vi "TDMS Strip Illegal Characters.vi"(5 "String":string) -> (2 "Legal String":string)   [LabVIEW 2011]
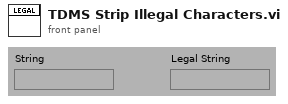
[diagram p1: front panel]
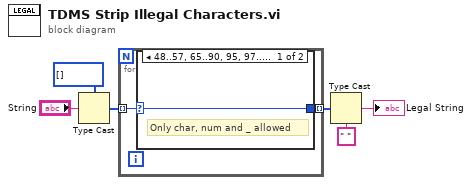
[diagram p0: block diagram]
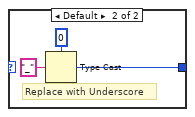
[diagram p2: hidden frame]
diagram:
  n1 = Type Cast(type=u8[] [], x="String") -> (*(type *) &x=w4:u8[])
  n2 = for {
    tunnel: w4 -> [w7] mode=indexing
    tunnel: [w8] -> w3 mode=indexing
    n3 = case shown="48..57, 65..90, 95, 97..122" w7 {
      selector: w7 -> [w9 _]
      tunnel: [w9 w10] -> w8
      frame 48..57, 65..90, 95, 97..122 {
        # "Only char, num and _ allowed"
      }
      frame Default {
        # "Replace with Underscore"
        n4 = Type Cast(type=u8 0, x="_") -> (*(type *) &x=w10:u8)
      }
    }
  }
  n5 = Type Cast(type=" ", x=w3) -> (*(type *) &x=→"Legal String":string)
